vi "Set Harmonic Multiplier.vi"(8 "error in (no error)":errorcluster, 10 "Harmonic Multiplier":i32, 11 "Handle in":i32) -> (0 "error out":errorcluster, 3 "Handle out":i32)   [LabVIEW 2013, in "Thorlabs_MC2000B.lvlib"]
doc: "Set Harmonic Multiplier applied to external reference frequency (1-15)."
uses:
  <instrlib>/Thorlabs_MC2000B/Thorlabs_MC2000B.lvlib
  Program Files/National Instruments/LabVIEW 2011/instr.lib/Thorlabs_MC2000B/Library/MC2000CommandLibWin64.dll
  <instrlib>/Thorlabs_MC2000B/Library/MC2000CommandLibWin32.dll
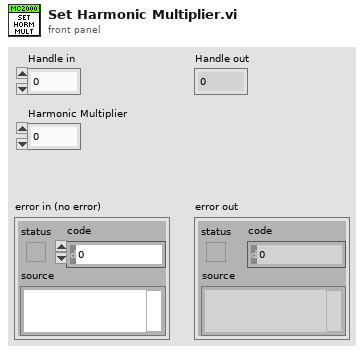
[diagram p1: front panel]
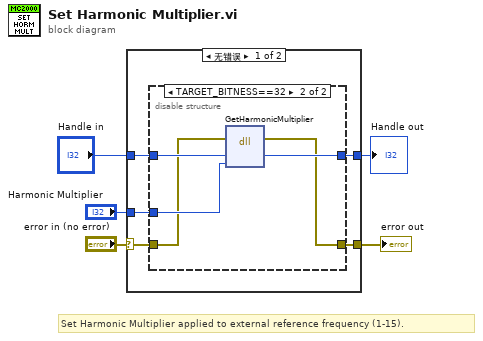
[diagram p0: block diagram]
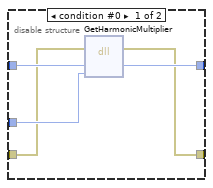
[diagram p2: hidden frame]
diagram:
  # "Set Harmonic Multiplier applied to external reference frequency (1-15)."
  n1 = case shown="无错误" "error in (no error)" {
    selector: "error in (no error)" -> [w7 w22]
    tunnel: [w6 w22] -> w5
    tunnel: "Harmonic Multiplier" -> [w8 _]
    tunnel: "Handle in" -> [w10 w21]
    tunnel: [w9 w21] -> w1
    frame No Error {
      n2 = disable-structure shown="TARGET_BITNESS==32" {
        disable-tunnel: w10 -> [w15 w20]
        disable-tunnel: [w14 w19] -> w9
        disable-tunnel: w8 -> [w13 w18]
        disable-tunnel: w7 -> [w12 w17]
        disable-tunnel: [w11 w16] -> w6
        frame condition #0 {
          n3 = dll-call lib="D:/Program Files/National Instruments/LabVIEW 2011/instr.lib/Thorlabs_MC2000B/Library/MC2000CommandLibWin64.dll" fn="GetHarmonicMultiplier"(error in=w12, "hdl"=w15, "nharmonic"=w13) -> (error out=w11:errorcluster, "hdl"=w14:i32)  [unwired: 4 in, 1 out]
        }
        frame condition #1 (active) {
          n4 = dll-call lib="C:/Program Files (x86)/National Instruments/LabVIEW 2013/instr.lib/Thorlabs_MC2000B/Library/MC2000CommandLibWin32.dll" fn="GetHarmonicMultiplier"(error in=w17, "hdl"=w20, "nharmonic"=w18) -> (error out=w16:errorcluster, "hdl"=w19:i32)  [unwired: 4 in, 1 out]
        }
      }
    }
    frame Error {
    }
  }
  "error out" <- w5
  "Handle out" <- w1
